vi "ACQ Start.vi"(8 "error in (no error)":errorcluster, 11 "VISA resource name In":T1={"Conection Data"="COM4"}) -> (0 "error out":errorcluster, 3 "VISA resource name Out":T1={"Conection Data"="COM4"})   [LabVIEW 2014, in "AD4212C Lib.lvlib"]
doc: "Detiene la adquisición de datos, limpia la UART y reinicia la adquisición."
uses:
  AD4212C Lib.lvlib
  Typedef/Connection Data.ctl
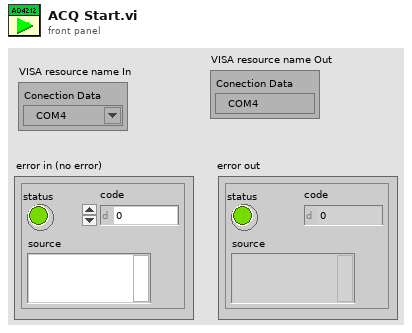
[diagram p1: front panel]
types:
  T1 = typedef "AD4212C Lib.lvlib/Connection Data.ctl" = cluster{"Conection Data":refnum<visa-resource-name>}
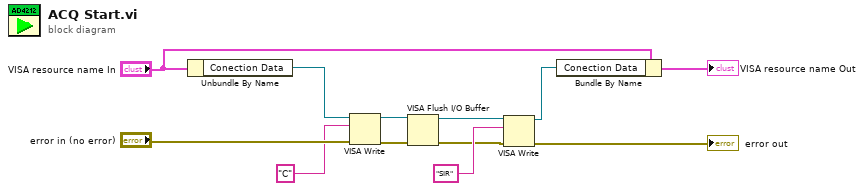
[diagram p0: block diagram]
diagram:
  n1 = Unbundle By Name("VISA resource name In") -> ("Conection Data"=w4:refnum<visa-resource-name>)
  n2 = VISA Write(VISA resource name=w4, write buffer="C", error in (no error)="error in (no error)") -> (VISA resource name out=w12:refnum<visa-resource-name>, error out=w6:errorcluster)  [unwired: 1 out]
  n3 = VISA Flush I/O Buffer(VISA resource name=w12, error in (no error)=w6) -> (VISA resource name out=w8:refnum<visa-resource-name>, error out=w5:errorcluster)  [unwired: 1 in]
  n4 = VISA Write(VISA resource name=w8, write buffer="SIR", error in (no error)=w5) -> (VISA resource name out=w3:refnum<visa-resource-name>, error out=→"error out":errorcluster)  [unwired: 1 out]
  n5 = Bundle By Name(cluster="VISA resource name In", "Conection Data"=w3) -> (→"VISA resource name Out":T1)
